vi "Write Stack Info.vi"(8 "error in (no error)":errorcluster, 10 "Stack Info":T1, 11 "Tiff Writer in":refnum<class "Tiff Writer.lvclass">) -> (0 "error out":errorcluster, 3 "Tiff Writer out":refnum<class "Tiff Writer.lvclass">)   [LabVIEW 2015, in "Tiff Writer.lvlib" / "Tiff Writer.lvclass"]
uses:
  Tiff Writer.lvclass
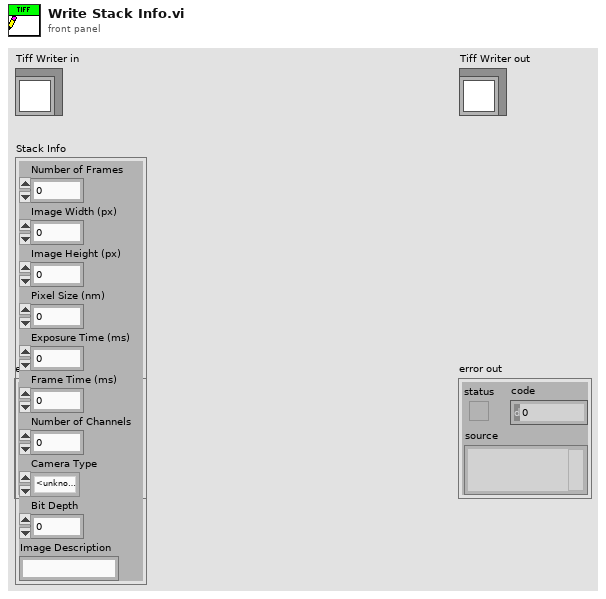
[diagram p1: front panel]
types:
  T1 = cluster{"Number of Frames":u32, "Image Width (px)":u32, "Image Height (px)":u32, "Pixel Size (nm)":dbl, "Exposure Time (ms)":dbl, "Frame Time (ms)":dbl, "Number of Channels":u32, "Camera Type":enum16{"<unknown>", "Evolve 512", "Orca-Flash 4.0 V2"}, "Bit Depth":u32, "Image Description":string}
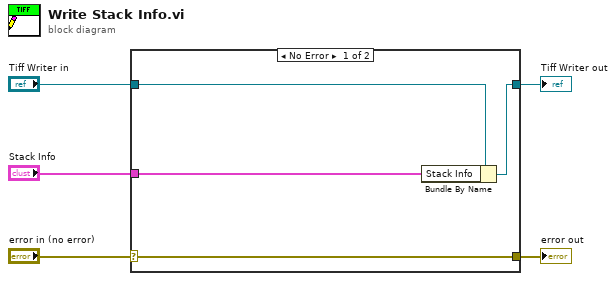
[diagram p0: block diagram]
diagram:
  n1 = case shown="No Error" "error in (no error)" {
    selector: "error in (no error)" -> [w9 w10]
    tunnel: [w9 w10] -> w4
    tunnel: [w7 w11] -> w2
    tunnel: "Tiff Writer in" -> [w8 w11]
    tunnel: "Stack Info" -> [w6 _]
    frame No Error {
      n2 = Bundle By Name(cluster=w8, "Stack Info"=w6) -> (w7:refnum<class "Tiff Writer.lvclass">)
    }
    frame Error {
    }
  }
  "error out" <- w4
  "Tiff Writer out" <- w2
